vi "Upload.vi"(5 "wait until completion? (T)":bool=TRUE, 6 "Delay Time (s)":dbl=0.5, 7 "DTR Delay":dbl=1.0, 8 "error in":errorcluster, 9 "Serial Port To Test":refnum<visa-resource-name>, 10 "working directory":path=path "C:/Users/TEDCAR~1/AppData/Local/Temp/AeroQuadFlightSoftware/AeroQuad", 11 "command line":string="cmd /c @echo Uploading flight software to microcontroller... & @ PATH=C:\\PROGRA~1\\ARDUIN~1.0\\hardware\\tools\\avr\\utils\\bin;%PATH% & cmd /c make sizeafter upload & pause") -> (0 "error out":errorcluster, 1 "Serial Port To Test Out":refnum<visa-resource-name>)   [LabVIEW 2010]
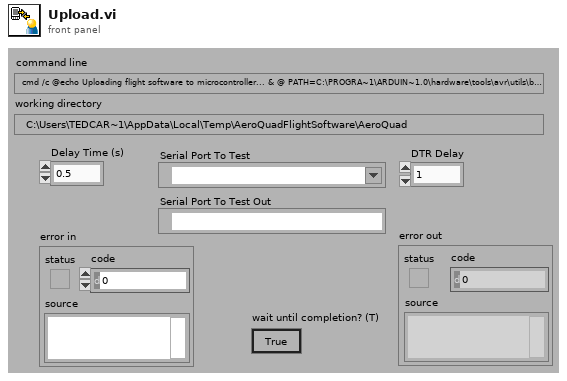
[diagram p1: front panel]
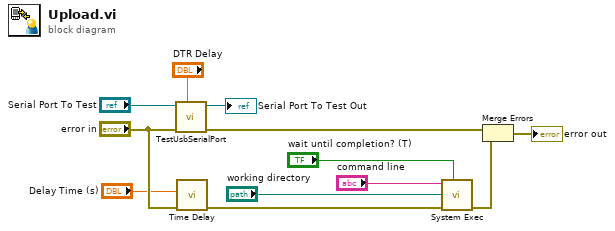
[diagram p0: block diagram]
diagram:
  n1 = call "TestUsbSerialPort.vi"("DTR Delay"="DTR Delay", "Error In"="error in", "Serial Port To Test"="Serial Port To Test") -> ("Error Out"=w10:errorcluster, "Output Serial Port"=→"Serial Port To Test Out":refnum<visa-resource-name>)  [unwired: 7 in]
  n2 = call "Time Delay"("error in (no error)"="error in", "Delay Time (s)"="Delay Time (s)") -> ("error out"=w6:errorcluster)  [unwired: 9 in]
  n3 = call <vilib>:"System Exec.vi"("wait until completion? (T)"="wait until completion? (T)", "error in (no error)"=w6, "working directory"="working directory", "command line"="command line") -> ("error out"=w9:errorcluster)  [unwired: 4 in, 3 out]
  n4 = Merge Errors(w10, w9) -> (→"error out":errorcluster)
